vi "Manufacturing-LoadSingleStep.vi"(8 "error in (no error)":errorcluster, 11 "ERP-CreateInstructions in":refnum<class "ERP-CreateInstructions.lvclass">) -> (0 "error out":errorcluster, 1 "Step#":i32, 3 "ERP-CreateInstructions out":refnum<class "ERP-CreateInstructions.lvclass">, 5 "Cluster for Step":T1, 7 "Part Number":string)   [LabVIEW 2013, in "ERP-CreateInstructions.lvclass"]
uses:
  ERP-CreateInstructions.lvclass
  ERP-CreateInstructions.lvclass/ERP-CreateInstructions.ctl
  <userlib>/_OpenG.lib/string/string.llb/Trim Whitespace (String Array)__ogtk.vi
  <userlib>/_OpenG.lib/array/array.llb/Search 1D Array (String)__ogtk.vi
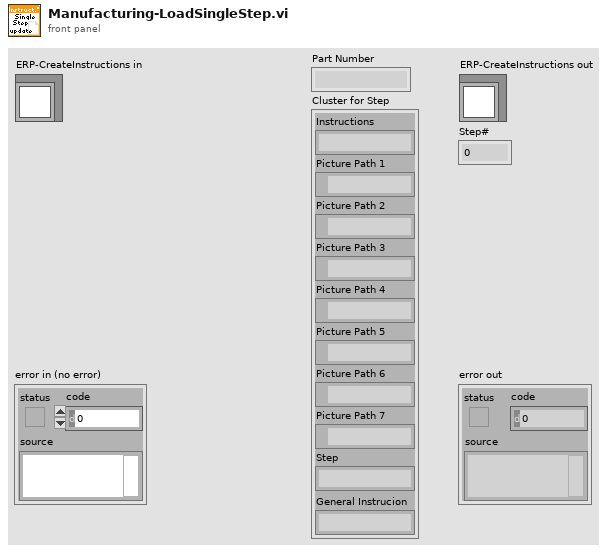
[diagram p1: front panel]
types:
  T1 = cluster{"Instructions":string, "Picture Path 1":path, "Picture Path 2":path, "Picture Path 3":path, "Picture Path 4":path, "Picture Path 5":path, "Picture Path 6":path, "Picture Path 7":path, "Step":string, "General Instrucion":string}
  T2 = cluster{"Instructions":string, "Picture Path 1":path, "Picture Path 2":path, "Picture Path 3":path, "Picture Path 4":path, "Picture Path 5":path, "Picture Path 6":path, "Picture Path 7":path, "Step":string, "General Instruction":string}
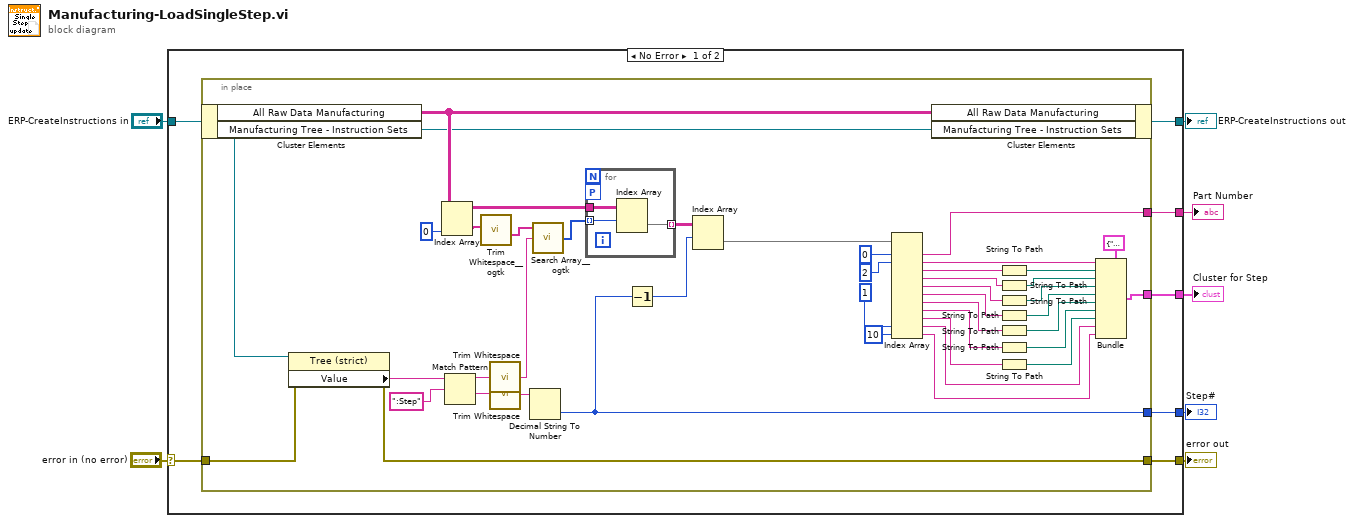
[diagram p0: block diagram]
diagram:
  n1 = case shown="No Error" "error in (no error)" {
    selector: "error in (no error)" -> [w12 w61]
    tunnel: [w10 w61] -> w6
    tunnel: [w13 w60] -> w4
    tunnel: "ERP-CreateInstructions in" -> [w14 w60]
    tunnel: [w11 _] -> w1
    tunnel: [w9 _] -> w3
    tunnel: [w8 _] -> w2
    frame No Error {
      n2 = in-place {
        in-place-border: w12 -> [w56]
        in-place-border: [w36] -> w11
        in-place-border: [w44] -> w10
        in-place-border: [w23] -> w9
        in-place-border: [w33] -> w8
        n3 = in-place-cluster #1(w14) -> ("All Raw Data Manufacturing"=w46:string[][], "Manufacturing Tree - Instruction Sets"=w45:refnum<vi>)
        n4 = property class="Tree (strict)"(reference=w45, error in=w56) -> (error out=w44:errorcluster, "Value"=w55:string)  [unwired: 1 out]
        n5 = Index Array(array=w46, index (col)=0 ("disabled index (col)")) -> (element=w26:string[])  [unwired: 1 in]
        n6 = Match Pattern(string=w55, regular expression=":Step") -> (before substring=w53:string, after substring=w52:string)  [unwired: 1 in, 2 out]
        n7 = call-poly <userlib>:"Trim Whitespace__ogtk.vi"("String in"=w26) -> ("String out"=w25:string[])  [unwired: 6 in]
        n8 = call <vilib>:"Trim Whitespace.vi"("string"=w53) -> ("trimmed string"=w49:string)  [unwired: 1 in]
        n9 = call <vilib>:"Trim Whitespace.vi"("string"=w52) -> ("trimmed string"=w50:string)  [unwired: 1 in]
        n10 = Decimal String To Number(string=w50) -> (number=w23:i32)  [unwired: 2 in, 1 out]
        n11 = call-poly <userlib>:"Search Array__ogtk.vi"("Array"=w25, "Element Data"=w49) -> ("Indices of Elements"=w48:i32[])  [unwired: 7 in]
        n12 = for {
          tunnel: w46 -> [w59]
          tunnel: w48 -> [w58] mode=indexing
          tunnel: [w57] -> w47 mode=indexing
          workers-P: _ -> [_]
          n13 = Index Array(array=w59, index (row)=w58) -> (element=w57:string[])  [unwired: 1 in]
        }
        n14 = Decrement(x=w23) -> (x-1=w24:i32)
        n15 = Index Array(array=w47, index (row)=w24) -> (element=w17:string[])  [unwired: 1 in]
        n16 = Index Array(array=w17, index #1=0 ("index"), index #2=2 ("index"), index #10=1 ("index"), index #11=10 ("index")) -> (element #1=w33:string, element #2=w35:string, element #3=w43:string, element #4=w42:string, element #5=w41:string, element #6=w40:string, element #7=w39:string, element #8=w38:string, element #9=w37:string, element #10=w18:string, element #11=w15:string)  [unwired: 7 in]
        n17 = in-place-cluster #1("All Raw Data Manufacturing"=w46, "Manufacturing Tree - Instruction Sets"=w45) -> (w13:refnum<class "ERP-CreateInstructions.lvclass">)
        n18 = String To Path(string=w43) -> (path=w34:path)
        n19 = String To Path(string=w42) -> (path=w32:path)
        n20 = String To Path(string=w41) -> (path=w31:path)
        n21 = String To Path(string=w40) -> (path=w30:path)
        n22 = String To Path(string=w39) -> (path=w29:path)
        n23 = String To Path(string=w38) -> (path=w28:path)
        n24 = String To Path(string=w37) -> (path=w27:path)
        n25 = Bundle(cluster=T2 {"Instructions"="", "Picture Path 1"=path "", "Picture Path 2"=path "", "Picture Path 3"=path "", "Picture Path 4"=path "", "Picture Path 5"=path "", "Picture Path 6"=path "", "Picture Path 7"=path "", "Step"="", "General Instruction"=""}, "Instructions"=w35, "Picture Path 1"=w34, "Picture Path 2"=w32, "Picture Path 3"=w31, "Picture Path 4"=w30, "Picture Path 5"=w29, "Picture Path 6"=w28, "Picture Path 7"=w27, "Step"=w18, "General Instruction"=w15) -> (w36:T2)
      }
    }
    frame Error {
    }
  }
  "error out" <- w6
  "ERP-CreateInstructions out" <- w4
  "Step#" <- w3
  "Part Number" <- w2
  "Cluster for Step" <- w1
